vi "Write Paths.vi"(8 "error in (no error)":errorcluster, 10 "Paths":T1[](array[typedef]), 11 "ParseXML in":refnum<class "ParseSVG.lvclass">) -> (0 "error out":errorcluster, 3 "ParseXML out":refnum<class "ParseSVG.lvclass">)   [LabVIEW 2019, in "ParseSVG.lvclass"]
uses:
  ParseSVG.lvclass
  Path.ctl
  ParseSVG.lvclass/ParseSVG.ctl
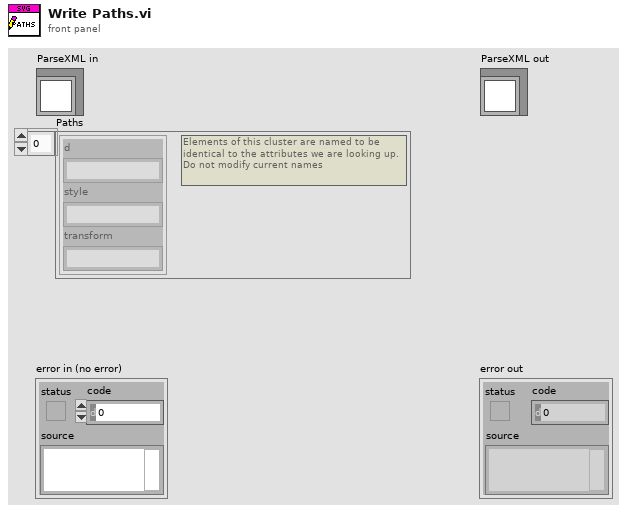
[diagram p1: front panel]
types:
  T1 = typedef "ParseSVG.lvclass/Path.ctl" = cluster{"d":string, "style":string, "transform":string}
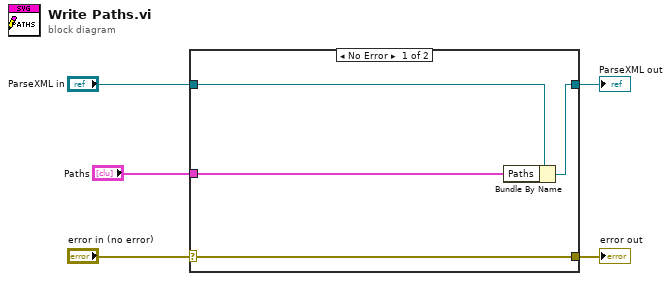
[diagram p0: block diagram]
diagram:
  n1 = case shown="No Error" "error in (no error)" {
    selector: "error in (no error)" -> [w9 w10]
    tunnel: [w9 w10] -> w4
    tunnel: [w7 w11] -> w2
    tunnel: "ParseXML in" -> [w8 w11]
    tunnel: "Paths" -> [w6 _]
    frame No Error {
      n2 = Bundle By Name(cluster=w8, "Paths"=w6) -> (w7:refnum<class "ParseSVG.lvclass">)
    }
    frame Error {
    }
  }
  "error out" <- w4
  "ParseXML out" <- w2
